vi "Init SPI CS.vi"(7 "CS GPIO":T1=5, 8 "error in (no error)":errorcluster, 10 "CS Active Low (T)":bool=TRUE, 11 "Session in":refnum<class "Session.lvclass">) -> (0 "error out":errorcluster, 2 "SPI CS":refnum<class "SPI CS.lvclass">, 3 "Session out":refnum<class "Session.lvclass">)   [LabVIEW 2020, in "CTI.lvlib" / "Session.lvclass"]
uses:
  Session.lvclass
  Session.lvclass/Session.ctl
  SPI CS/SPI CS.lvclass
  GPIO Number.ctl
  CTI.lvlib
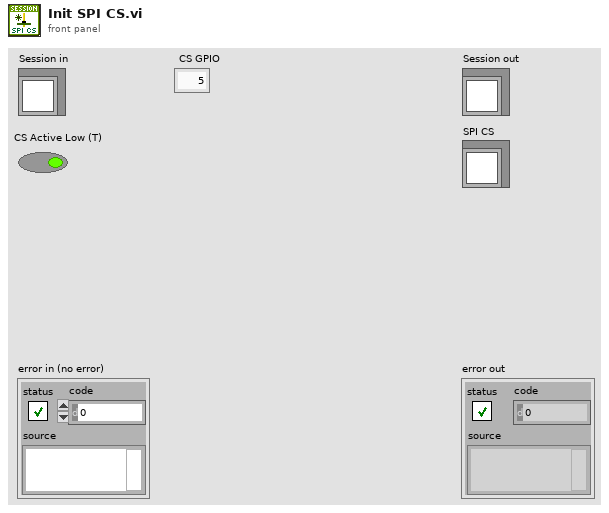
[diagram p1: front panel]
types:
  T1 = typedef "CTI.lvlib/GPIO Number.ctl" = i8
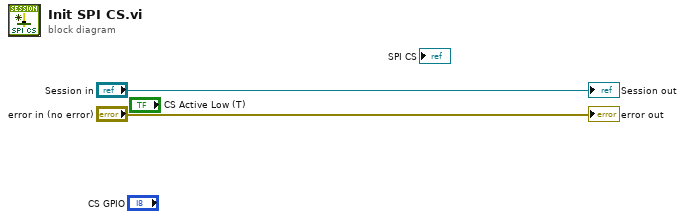
[diagram p0: block diagram]
diagram:
  "error out" <- "error in (no error)"
  "Session out" <- "Session in"
